vi "Conveyor.vi"() -> ()   [LabVIEW 2021]
panel:
  out "Boolean 2":bool
  out "Boolean":bool
  in  "Conveyor Keripik 2":dbl(slide) scale=0.0..10.0
  in  "Conveyor Keripik":dbl(slide) scale=0.0..10.0
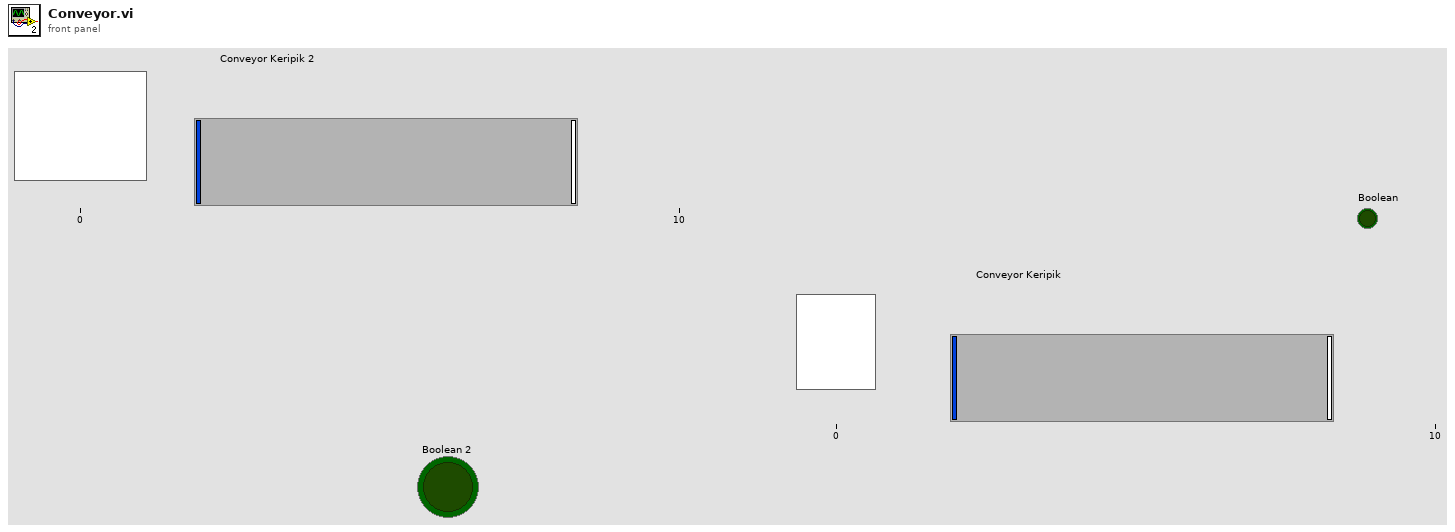
[diagram p1: front panel]
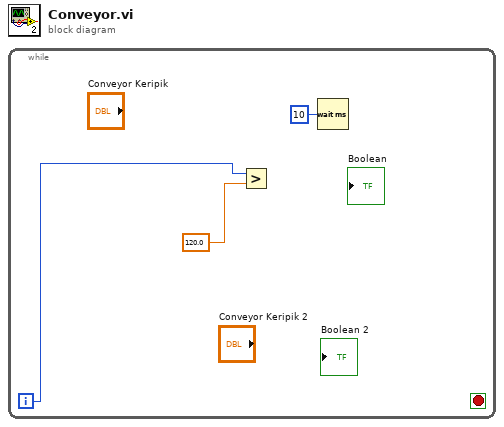
[diagram p0: block diagram]
diagram:
  n1 = while {
    i -> [w1]
    stop <- w2 stop-if-true
    n2 = Greater?(x=w1, y=120.0) -> ()  [unwired: 1 out]
    n3 = Wait (ms)(milliseconds to wait=u32 10) -> ()  [unwired: 1 out]
  }
